vi "Get Shape.vi"(11 "Particle in":refnum<class "Particle.lvclass">) -> (1 "Color":u32(colorbox), 2 "Coordinates":cluster{"X":i32, "Y":i32}[](array[cluster]), 3 "Particle out":refnum<class "Particle.lvclass">)   [LabVIEW 2020, in "Particle.lvclass"]
uses:
  Particle.lvclass
  Particle.lvclass/Particle.ctl
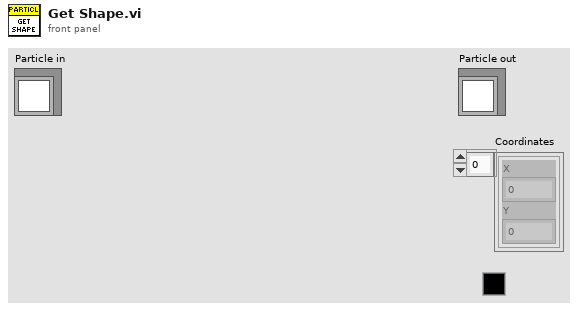
[diagram p1: front panel]
types:
  T1 = typedef "Particle.lvclass/Position.ctl" = cluster{"X":i32, "Y":i32}
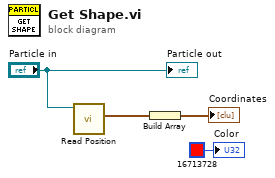
[diagram p0: block diagram]
diagram:
  n1 = call "Read Position.vi"("Particle in"="Particle in") -> ("Position"=w2:T1)  [unwired: 10 in]
  n2 = Build Array(w2) -> (→"Coordinates":T1[])
  "Particle out" <- "Particle in"
  "Color" <- u32 16713728 ("Color")
